vi "print console2.vi"() -> ()   [LabVIEW 2018]
doc: "이 템플릿을 사용하여 이벤트와 함께 큐 아이템을 생성하는 생산자/소비자 디자인 패턴을 생성합니다. 사용자 인터페이스의 반응을 느리게 하지 않고 이벤트에 대응하여 비동기적으로 코드를 실행시키려고 할 때, 사용자 인터페이스의 이벤트 핸들러 패턴 대신에 이 디자인 패턴을 사용하십시오."
panel:
  in  "Enqueue Element":bool caption="원소를 큐에 추가"
  in  "stop":bool caption="정지"
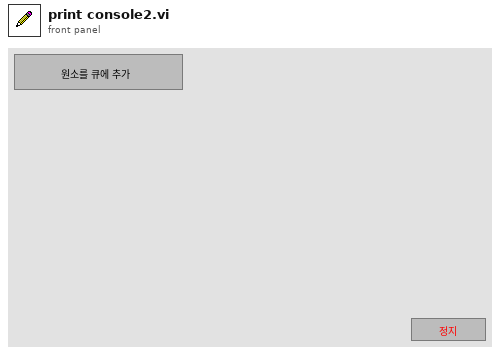
[diagram p1: front panel]
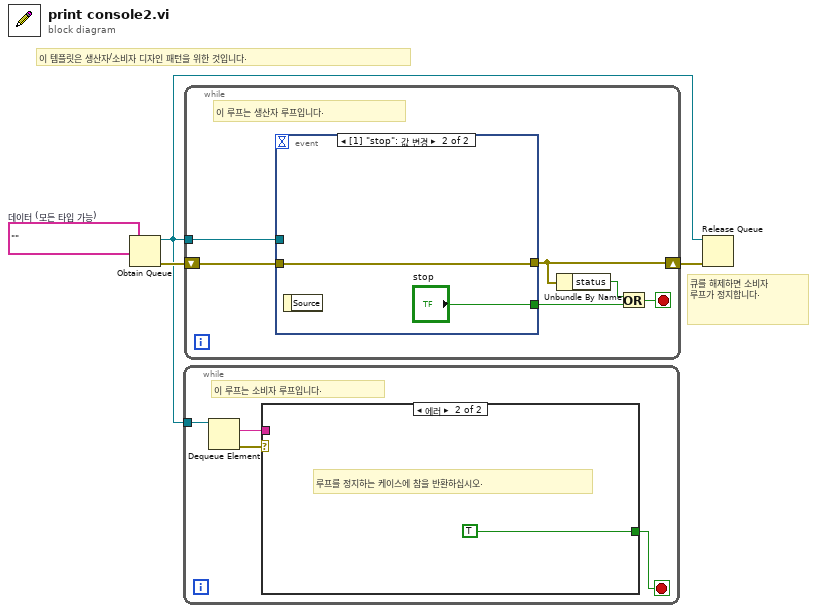
[diagram p0: block diagram]
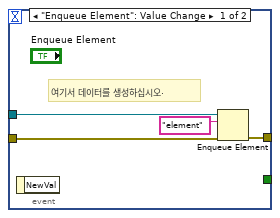
[diagram p3: hidden frame]
diagram:
  w2 = ""  # 데이터 (모든 타입 가능)
  # "큐를 해제하면 소비자 루프가 정지합니다."
  # "이 템플릿은 생산자/소비자 디자인 패턴을 위한 것입니다."
  n1 = Obtain Queue(element data type=w2) -> (queue out=w1:refnum<queue>, error out=w4:errorcluster)  [unwired: 4 in, 1 out]
  n2 = while {
    tunnel: w1 -> [w8]
    stop <- w5 stop-if-true
    # "이 루프는 소비자 루프입니다."
    n3 = Dequeue Element(queue=w8) -> (element=w6:string, error out=w7:errorcluster)  [unwired: 2 in, 2 out]
    n4 = case shown="에러" w7 {
      tunnel: w6 -> [_ _]
      tunnel: [_ TRUE] -> w5
      frame No Error {
        # "여기서 데이터를 처리하십시오."
      }
      frame Error {
        # "루프를 정지하는 케이스에 참을 반환하십시오."
      }
    }
  }
  n5 = while {
    shift-right: [w11] -> w3
    shift-left: w4 -> [w14]
    tunnel: w1 -> [w15]
    stop <- w12 stop-if-true
    # "이 루프는 생산자 루프입니다."
    n6 = event shown="[1] \"stop\": 값 변경" {
      selector: _ -> [_ _]
      dyn-events: _ -> [_ _]
      timeout: _ -> [_ _]
      tunnel: w15 -> [w19 _]
      tunnel: w14 -> [w18 w20]
      tunnel: [w17 w20] -> w11
      tunnel: [_ "stop"] -> w13
      event "Enqueue Element": Value Change {
        # "여기서 데이터를 생성하십시오."
        n7 = event-data() -> ()  [unwired: 1 in, 1 out]
        n8 = Enqueue Element(queue=w19, element="element", error in (no error)=w18) -> (error out=w17:errorcluster)  [unwired: 1 in, 2 out]
      }
      event "stop": Value Change {
        n9 = event-data() -> ()  [unwired: 1 in, 1 out]
      }
    }
    n10 = Unbundle By Name(w11) -> ("status"=w10:bool)
    n11 = Or(x=w10, y=w13) -> (x .or. y?=w12:bool)
  }
  n12 = Release Queue(queue=w1, error in (no error)=w3) -> ()  [unwired: 1 in, 3 out]
